vi "LWXPS_TZMotorDecouplingMatrixGet.vi"(0 "XPS Reference IN":refnum<k24>, 2 "Group Name":string, 5 "LabVIEW error IN":errorcluster) -> (7 "LabVIEW error OUT":errorcluster, 8 "XPS Reference OUT":refnum<k24>, 9 "XPS Error String":string, 10 "Returned error code":i32, 11 "Value 3 3":dbl, 12 "Value 1 1":dbl, 13 "Value 3 2":dbl, 14 "Value 1 2":dbl, 15 "Value 1 3":dbl, 16 "Value 2 1":dbl, 17 "Value 2 2":dbl, 18 "Value 2 3":dbl, 19 "Value 3 1":dbl)   [LabVIEW 2014]
uses:
  D:/XPSQ8_LabView_Library/Development/Source/Dll/Newport.XPS.CommandInterface.dll
  Dll/Newport.XPS.CommandInterface.dll
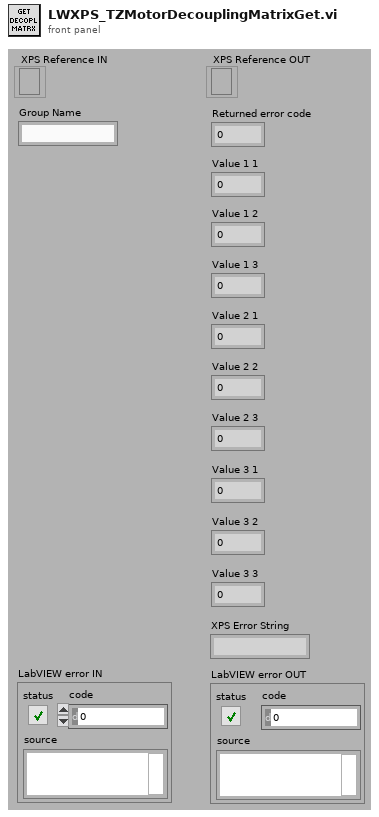
[diagram p1: front panel]
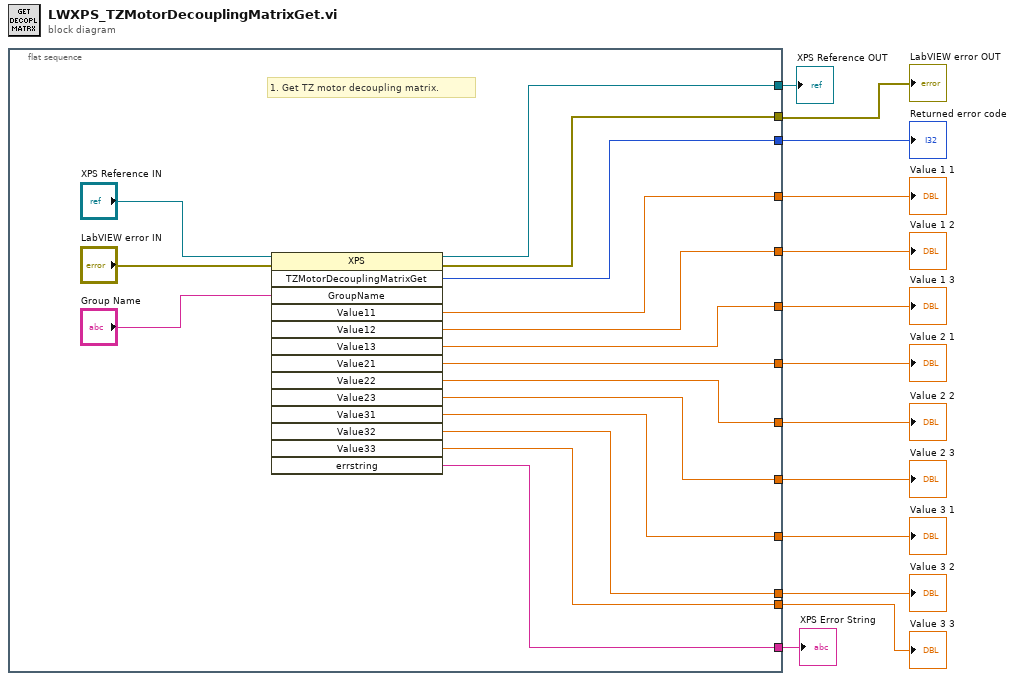
[diagram p0: block diagram]
diagram:
  n1 = flat-sequence {
    tunnel: [w27] -> w13
    tunnel: [w25] -> w12
    tunnel: [w28] -> w11
    tunnel: [w20] -> w2
    tunnel: [w23] -> w10
    tunnel: [w24] -> w7
    tunnel: [w22] -> w9
    tunnel: [w21] -> w8
    tunnel: [w19] -> w6
    tunnel: [w18] -> w5
    tunnel: [w17] -> w4
    tunnel: [w16] -> w3
    tunnel: [w15] -> w1
    frame #0 {
      # "1. Get TZ motor decoupling matrix."
      n2 = invoke class="XPS" method="TZMotorDecouplingMatrixGet"(reference="XPS Reference IN", error in="LabVIEW error IN", "GroupName"="Group Name") -> (reference out=w27:refnum<k24>, error out=w25:errorcluster, "TZMotorDecouplingMatrixGet"=w28:i32, "Value11"=w20:dbl, "Value12"=w23:dbl, "Value13"=w22:dbl, "Value21"=w21:dbl, "Value22"=w24:dbl, "Value23"=w19:dbl, "Value31"=w18:dbl, "Value32"=w17:dbl, "Value33"=w16:dbl, "errstring"=w15:string)  [unwired: 11 in, 1 out]
    }
  }
  "XPS Error String" <- w1
  "XPS Reference OUT" <- w13
  "LabVIEW error OUT" <- w12
  "Returned error code" <- w11
  "Value 1 2" <- w10
  "Value 1 3" <- w9
  "Value 2 1" <- w8
  "Value 2 2" <- w7
  "Value 2 3" <- w6
  "Value 3 1" <- w5
  "Value 3 2" <- w4
  "Value 3 3" <- w3
  "Value 1 1" <- w2
